vi "StartEstablishHome.vi"(8 "error in (no error)":errorcluster, 11 "VXMMotionManager in":refnum<class "VXMMotionManager.lvclass">) -> (0 "error out":errorcluster, 3 "VXMMotionManager out":refnum<class "VXMMotionManager.lvclass">)   [LabVIEW 2019, in "VXMMotionManager.lvclass"]
doc: "Load up properties for a sequence of motion that finds all four home positions, zeros counters"
uses:
  VXMMotionManager.lvclass
  MoveAllAbsoluteStates.ctl
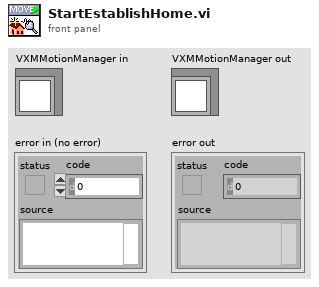
[diagram p1: front panel]
types:
  T1 = typedef "VXMMotionManager.lvclass/MoveAllAbsoluteStates.ctl" = enum16{"start next move", "wait motion end"}
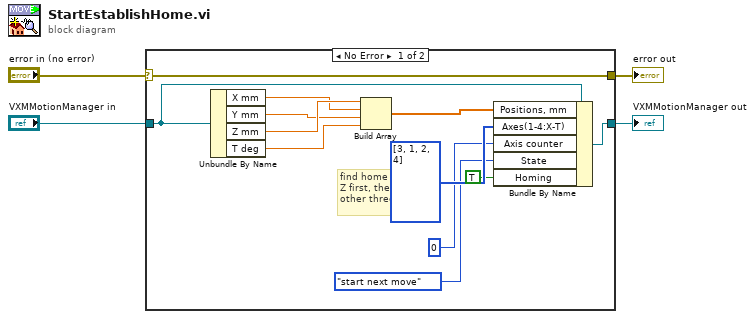
[diagram p0: block diagram]
diagram:
  n1 = case shown="No Error" "error in (no error)" {
    selector: "error in (no error)" -> [w16 w18]
    tunnel: [w16 w18] -> w3
    tunnel: [w15 w17] -> w1
    tunnel: "VXMMotionManager in" -> [w11 w17]
    frame No Error {
      # "find home for \nZ first, then\nother three"
      n2 = Unbundle By Name(w11) -> ("X mm"=w9:dbl, "Y mm"=w8:dbl, "Z mm"=w10:dbl, "T deg"=w7:dbl)
      n3 = Build Array(w10, w9, w8, w7) -> (w6:dbl[])
      n4 = Bundle By Name(cluster=w11, "Positions, mm"=w6, "Axes(1-4:X-T)"=i32[] [3, 1, 2, 4], "Axis counter"=0, "State"=MoveAllAbsoluteStates."start next move", "Homing"=TRUE) -> (w15:refnum<class "VXMMotionManager.lvclass">)
    }
    frame Error {
    }
  }
  "error out" <- w3
  "VXMMotionManager out" <- w1
